vi "HEIGHT CONTROL ORNL Ver1.vi"() -> ()   [LabVIEW 2016]
panel:
  out "Beads":T1
  in  "stop":bool
  in  "Decimation":dbl=10.0 format="%#_13g"
  out "Print/Scan":bool
  out "Bead Profiles":cluster{dbl[], dbl[]}[](graph)
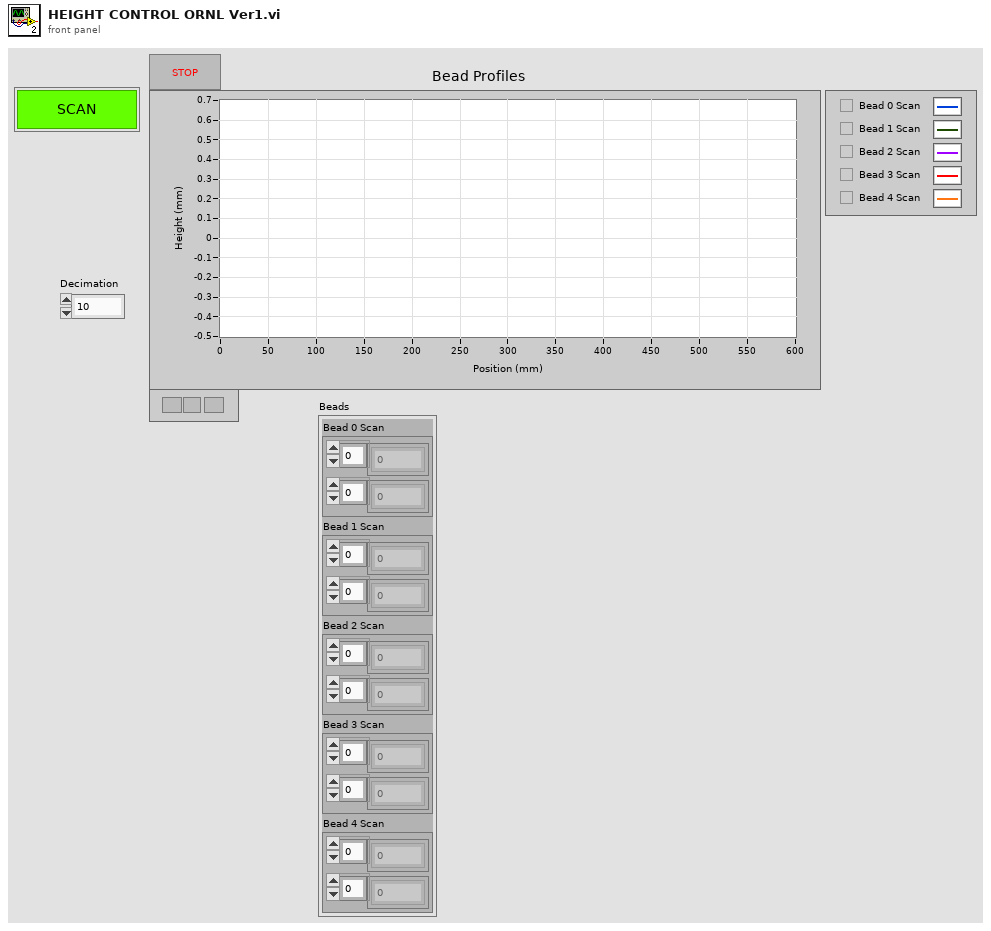
[diagram p1: front panel]
types:
  T1 = cluster{"Bead 0 Scan":cluster{dbl[], dbl[]}, "Bead 1 Scan":cluster{dbl[], dbl[]}, "Bead 2 Scan":cluster{dbl[], dbl[]}, "Bead 3 Scan":cluster{dbl[], dbl[]}, "Bead 4 Scan":cluster{dbl[], dbl[]}}
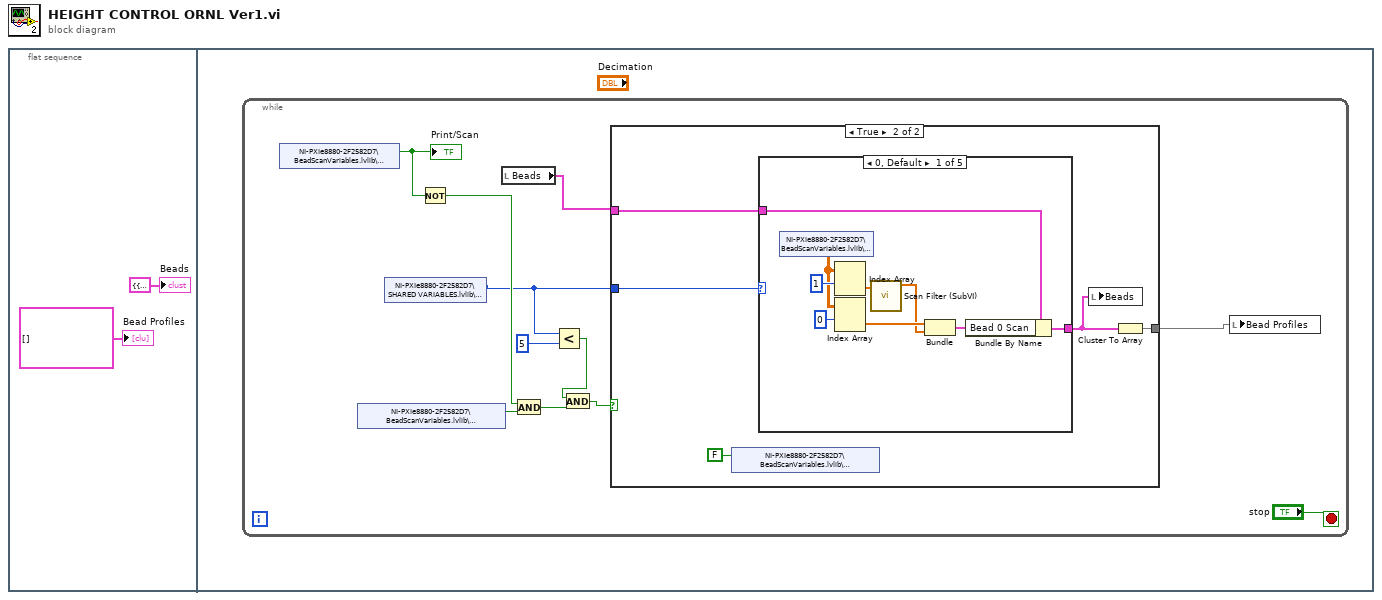
[diagram p0: block diagram]
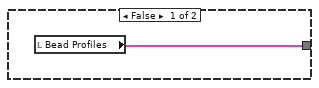
[diagram p2: hidden frame]
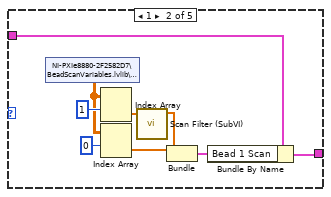
[diagram p3: hidden frame]
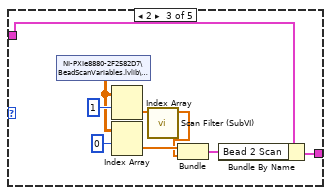
[diagram p4: hidden frame]
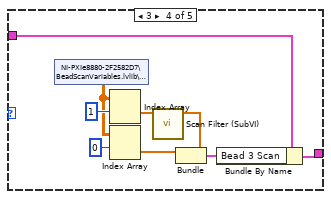
[diagram p5: hidden frame]
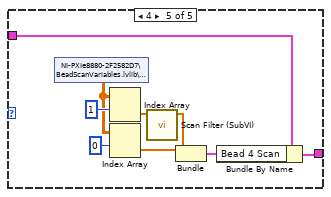
[diagram p6: hidden frame]
diagram:
  n1 = flat-sequence {
    frame #0 {
      "Beads" <- T1 {"Bead 0 Scan"={[], []}, "Bead 1 Scan"={[], []}, "Bead 2 Scan"={[], []}, "Bead 3 Scan"={[], []}, "Bead 4 Scan"={[], []}} ("Beads")
      "Bead Profiles" <- cluster{dbl[], dbl[]}[] [] ("Bead Profiles")
    }
    frame #1 {
      n2 = while {
        stop <- "stop" stop-if-true
        n3 = shared-variable "NI-PXIe8880-2F2582D7\\BeadScanVariables.lvlib\\PRINTorSCAN"() -> (w11:bool)  [unwired: 1 in, 1 out]
        "Print/Scan" <- w11
        n4 = shared-variable "NI-PXIe8880-2F2582D7\\BeadScanVariables.lvlib\\BeadScanComplete"() -> (w12:bool)  [unwired: 1 in, 1 out]
        n5 = shared-variable "NI-PXIe8880-2F2582D7\\SHARED VARIABLES.lvlib\\Kuka Code"() -> (w9:u32)  [unwired: 1 in, 1 out]
        n6 = Not(x=w11) -> (.not. x?=w10:bool)
        n7 = local read "Beads"() -> (w4:T1)
        n8 = And(x=w10, y=w12) -> (x .and. y?=w7:bool)
        n9 = Less?(x=w9, y=u32 5) -> (x < y?=w6:bool)
        n10 = And(x=w6, y=w7) -> (x .and. y?=w5:bool)
        n11 = case shown="True" w5 {
          tunnel: [w14 w19] -> w3
          tunnel: w9 -> [_ w18]
          tunnel: w4 -> [_ w17]
          frame False {
            n12 = local read "Bead Profiles"() -> (w14:cluster{dbl[], dbl[]}[])
          }
          frame True {
            n13 = shared-variable "NI-PXIe8880-2F2582D7\\BeadScanVariables.lvlib\\BeadScanComplete"(FALSE ("BeadScanComplete")) -> ()  [unwired: 1 in, 1 out]
            n14 = case shown="0, Default" w18 {
              tunnel: w17 -> [w24 w31 w41 w50 w58]
              tunnel: [w23 w32 w40 w49 w59] -> w16
              frame 0, Default {
                n15 = shared-variable "NI-PXIe8880-2F2582D7\\BeadScanVariables.lvlib\\ScanData"() -> (w25:dbl[][])  [unwired: 1 in, 1 out]
                n16 = Index Array(array=w25, index (row)=1) -> (element=w22:dbl[])  [unwired: 1 in]
                n17 = Index Array(array=w25, index (row)=0) -> (element=w26:dbl[])  [unwired: 1 in]
                n18 = call "Scan Filter (SubVI).vi"("Array in"=w22) -> ("Array out"=w20:dbl[])  [unwired: 10 in]
                n19 = Bundle(w26, "Array out"=w20) -> (w21:cluster{dbl[], "Array out":dbl[]})  [unwired: 1 in]
                n20 = Bundle By Name(cluster=w24, "Bead 0 Scan"=w21) -> (w23:T1)
              }
              frame 1 {
                n21 = shared-variable "NI-PXIe8880-2F2582D7\\BeadScanVariables.lvlib\\ScanData"() -> (w34:dbl[][])  [unwired: 1 in, 1 out]
                n22 = Index Array(array=w34, index (row)=1) -> (element=w30:dbl[])  [unwired: 1 in]
                n23 = Index Array(array=w34, index (row)=0) -> (element=w35:dbl[])  [unwired: 1 in]
                n24 = call "Scan Filter (SubVI).vi"("Array in"=w30) -> ("Array out"=w29:dbl[])  [unwired: 10 in]
                n25 = Bundle(w35, "Array out"=w29) -> (w33:cluster{dbl[], "Array out":dbl[]})  [unwired: 1 in]
                n26 = Bundle By Name(cluster=w31, "Bead 1 Scan"=w33) -> (w32:T1)
              }
              frame 2 {
                n27 = shared-variable "NI-PXIe8880-2F2582D7\\BeadScanVariables.lvlib\\ScanData"() -> (w43:dbl[][])  [unwired: 1 in, 1 out]
                n28 = Index Array(array=w43, index (row)=1) -> (element=w39:dbl[])  [unwired: 1 in]
                n29 = Index Array(array=w43, index (row)=0) -> (element=w44:dbl[])  [unwired: 1 in]
                n30 = call "Scan Filter (SubVI).vi"("Array in"=w39) -> ("Array out"=w38:dbl[])  [unwired: 10 in]
                n31 = Bundle(w44, "Array out"=w38) -> (w42:cluster{dbl[], "Array out":dbl[]})  [unwired: 1 in]
                n32 = Bundle By Name(cluster=w41, "Bead 2 Scan"=w42) -> (w40:T1)
              }
              frame 3 {
                n33 = shared-variable "NI-PXIe8880-2F2582D7\\BeadScanVariables.lvlib\\ScanData"() -> (w52:dbl[][])  [unwired: 1 in, 1 out]
                n34 = Index Array(array=w52, index (row)=1) -> (element=w48:dbl[])  [unwired: 1 in]
                n35 = Index Array(array=w52, index (row)=0) -> (element=w53:dbl[])  [unwired: 1 in]
                n36 = call "Scan Filter (SubVI).vi"("Array in"=w48) -> ("Array out"=w47:dbl[])  [unwired: 10 in]
                n37 = Bundle(w53, "Array out"=w47) -> (w51:cluster{dbl[], "Array out":dbl[]})  [unwired: 1 in]
                n38 = Bundle By Name(cluster=w50, "Bead 3 Scan"=w51) -> (w49:T1)
              }
              frame 4 {
                n39 = shared-variable "NI-PXIe8880-2F2582D7\\BeadScanVariables.lvlib\\ScanData"() -> (w61:dbl[][])  [unwired: 1 in, 1 out]
                n40 = Index Array(array=w61, index (row)=1) -> (element=w57:dbl[])  [unwired: 1 in]
                n41 = Index Array(array=w61, index (row)=0) -> (element=w62:dbl[])  [unwired: 1 in]
                n42 = call "Scan Filter (SubVI).vi"("Array in"=w57) -> ("Array out"=w56:dbl[])  [unwired: 10 in]
                n43 = Bundle(w62, "Array out"=w56) -> (w60:cluster{dbl[], "Array out":dbl[]})  [unwired: 1 in]
                n44 = Bundle By Name(cluster=w58, "Bead 4 Scan"=w60) -> (w59:T1)
              }
            }
            n45 = local write "Beads"(w16) -> ()
            n46 = Cluster To Array(cluster=w16) -> (array=w19:cluster{dbl[], dbl[]}[])
          }
        }
        n47 = local write "Bead Profiles"(w3) -> ()
      }
    }
  }
